vi "LLB Pre-Build CHM Build.vi"(6 "Top Level/Always Included VIs":path[](array[path]), 7 "Main Destination Path":path, 9 "Target Name":string, 10 "Build Specification Name":string, 11 "Project Path":path) -> (0 "error out":errorcluster)   [LabVIEW 2017]
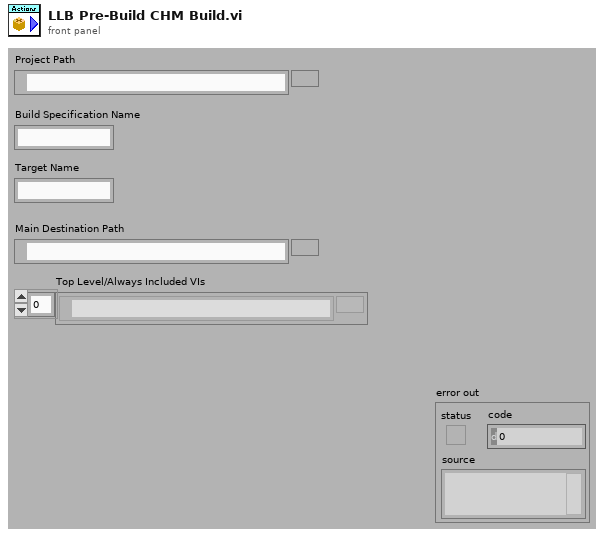
[diagram p1: front panel]
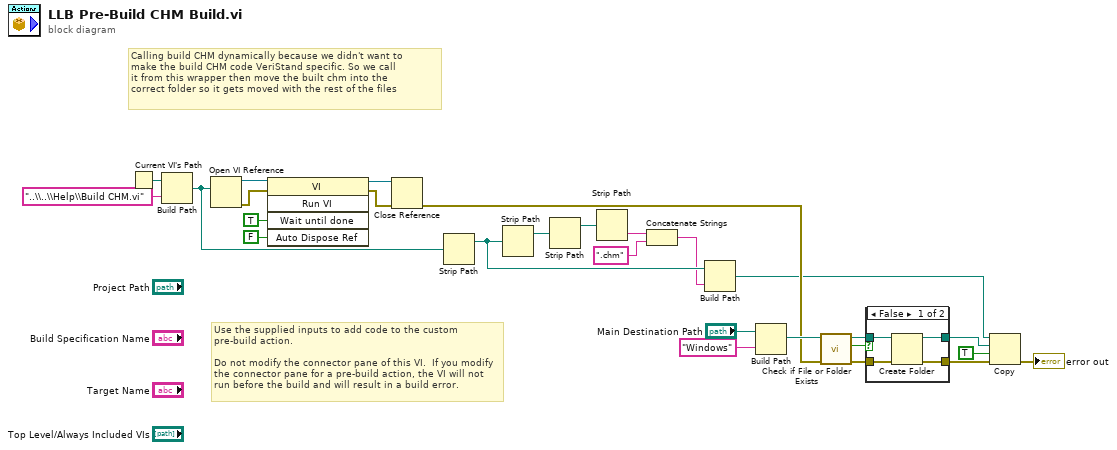
[diagram p0: block diagram]
diagram:
  # "Calling build CHM dynamically because we didn't want to \nmake the build CHM code VeriStand specific. So we call\nit from this wrapper then move the built chm into the\ncorrect folder so it gets moved with the rest of the files"
  # "Use the supplied inputs to add code to the custom pre-build action.\n\nDo not modify the connector pane of this VI.  If you modify the connector pane for a pre-build action, the VI will not run before the build and will result in a build error."
  n1 = Current VI's Path() -> (path=w27:path)
  n2 = Build Path(base path=w27, name or relative path="..\\..\\Help\\Build CHM.vi") -> (appended path=w19:path)
  n3 = Open VI Reference(vi path=w19) -> (vi reference=w25:refnum<vi>, error out=w24:errorcluster)  [unwired: 5 in]
  n4 = invoke class="VI" method="Run VI"(reference=w25, error in=w24, "Wait until done"=TRUE ("Wait Until Done"), "Auto Dispose Ref"=FALSE ("Auto Dispose Reference")) -> (reference out=w21:refnum<vi>, error out=w20:errorcluster)  [unwired: 1 in, 3 out]
  n5 = Close Reference(reference=w21, error in (no error)=w20) -> (error out=w9:errorcluster)
  n6 = Strip Path(path=w19) -> (stripped path=w18:path)  [unwired: 1 out]
  n7 = Strip Path(path=w18) -> (stripped path=w17:path)  [unwired: 1 out]
  n8 = Strip Path(path=w17) -> (stripped path=w16:path)  [unwired: 1 out]
  n9 = Strip Path(path=w16) -> (name=w15:string)  [unwired: 1 out]
  n10 = Concatenate Strings(w15, ".chm" ("string")) -> (w13:string)
  n11 = Build Path(base path=w18, name or relative path=w13) -> (appended path=w2:path)
  n12 = Build Path(base path="Main Destination Path", name or relative path="Windows") -> (appended path=w10:path)
  n13 = call <vilib>:"Check if File or Folder Exists.vi"("error in (no error)"=w9, "path"=w10) -> ("error out"=w6:errorcluster, "file or folder exists?"=w8:bool, "dup path"=w7:path)  [unwired: 7 in]
  n14 = case shown="False" w8 {
    tunnel: w7 -> [w30 w33]
    tunnel: w6 -> [w31 w32]
    tunnel: [w29 w33] -> w4
    tunnel: [w28 w32] -> w5
    frame False {
      n15 = Create Folder(path (use dialog)=w30, error in=w31) -> (created path=w29:path, error out=w28:errorcluster)  [unwired: 1 in, 1 out]
    }
    frame True {
    }
  }
  n16 = Copy(8:w5, 9:TRUE ("overwrite (F)"), 10:w4, 11:w2) -> (0:→"error out":errorcluster)  [unwired: 1 in, 2 out]
